vi "Bundle Message.vi"(7 "Amplitude":dbl format="%#_3g", 8 "Stage Number":string, 9 "Previous Position":i16, 10 "Position Threshold":i16, 11 "Current Position":i16) -> (1 "Output to queue":T1, 2 "Output Position":i16, 3 "Transition?":bool)   [LabVIEW 2016]
doc: "This VI checks if the current encoder position has passed the threshold for the current stage, and if so will set the Transition Boolean indicator to true. It also bundles position, amplitude, and the stage number string to add to the queue. The consumer loop will then take this information and write the LCD text accordingly."
uses:
  controls/Queue Data.ctl
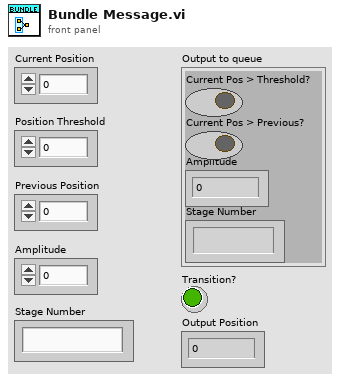
[diagram p1: front panel]
types:
  T1 = typedef "Queue Data.ctl" = cluster{"Current Pos > Threshold?":bool, "Current Pos > Previous?":bool, "Amplitude":dbl, "Stage Number":string}
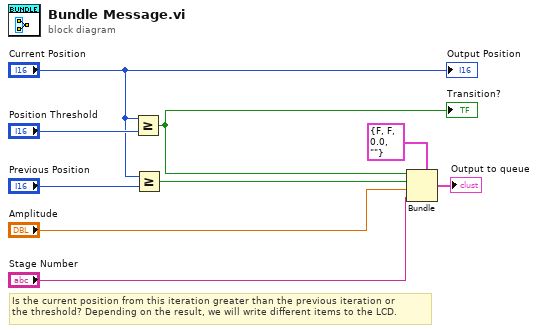
[diagram p0: block diagram]
diagram:
  # "Is the current position from this iteration greater than the previous iteration or\nthe threshold? Depending on the result, we will write different items to the LCD."
  n1 = Greater Or Equal?(x="Current Position", y="Position Threshold") -> (x >= y?=w2:bool)
  "Transition?" <- w2
  n2 = Greater Or Equal?(x="Current Position", y="Previous Position") -> (x >= y?=w8:bool)
  n3 = Bundle(cluster=T1 {"Current Pos > Threshold?"=FALSE, "Current Pos > Previous?"=FALSE, "Amplitude"=0.0, "Stage Number"=""} ("output to queue"), "Current Pos > Threshold?"=w2, "Current Pos > Previous?"=w8, "Amplitude"="Amplitude", "Stage Number"="Stage Number") -> (→"Output to queue":T1)
  "Output Position" <- "Current Position"
